vi "Math-Remove Group Delay.vi"(0 "Frequency (Hz)":dbl[](array[numeric]), 5 "Phase (cycles)":dbl[](array[numeric]), 9 "Fmax (Hz)":dbl=inf) -> (4 "Group Delay (ms)":dbl, 6 "Phase (cycles)":dbl[](array[numeric]))   [LabVIEW 2015]
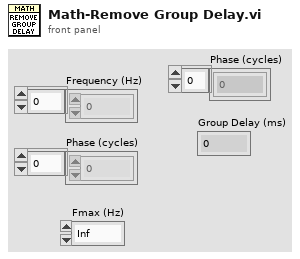
[diagram p1: front panel]
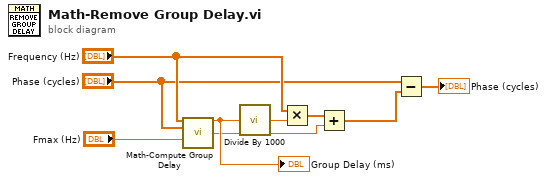
[diagram p0: block diagram]
diagram:
  n1 = call "Math-Compute Group Delay.vi"("Frequency (Hz)"="Frequency (Hz)", "Phase (cycles)"="Phase (cycles)", "Fmax (Hz)"="Fmax (Hz)") -> ("Group Delay (ms)"=w8:dbl, "Intercept (cycles)"=w4:dbl)  [unwired: 11 in]
  "Group Delay (ms)" <- w8
  n2 = call "Divide By 1000.vi"("X"=w8) -> ("X/1000"=w7:dbl)
  n3 = Multiply(x="Frequency (Hz)", y=w7) -> (x*y=w5:dbl[])
  n4 = Add(x=w5, y=w4) -> (x+y=w2:dbl[])
  n5 = Subtract(x="Phase (cycles)", y=w2) -> (x-y=→"Phase (cycles)":dbl[])
